vi "XY Graph Defer Owning VI Panel Update & Hide.vi"(6 "Defer Owning Panel Update":bool, 8 "error in (no error)":errorcluster, 11 "XY Graph Refnum in":refnum<vi>) -> (0 "error out":errorcluster, 3 "XY Graph Refnum out":refnum<vi>)   [LabVIEW 2019]
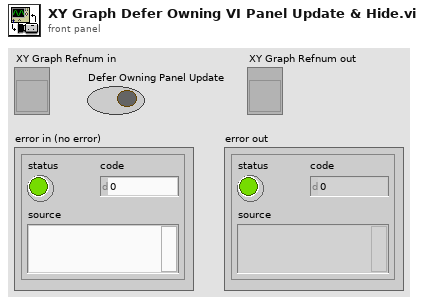
[diagram p1: front panel]
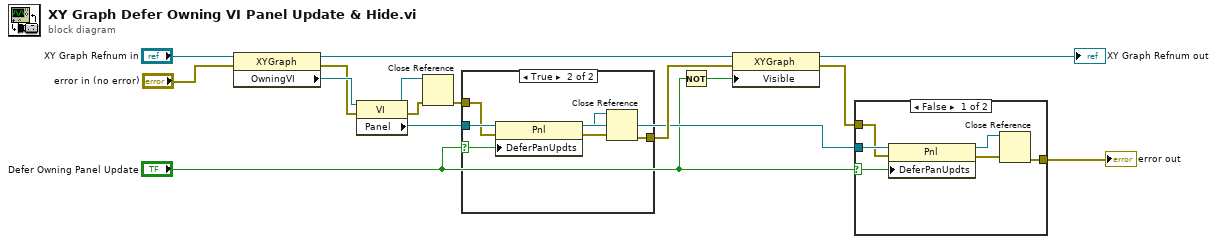
[diagram p0: block diagram]
diagram:
  n1 = property class="XYGraph"(reference="XY Graph Refnum in", error in="error in (no error)") -> (reference out=w13:refnum<vi>, error out=w3:errorcluster, "OwningVI"=w12:refnum<vi>)
  n2 = property class="VI"(reference=w12, error in=w3) -> (reference out=w11:refnum<vi>, error out=w10:errorcluster, "Panel"=w6:refnum<vi>)
  n3 = Close Reference(reference=w11, error in (no error)=w10) -> (error out=w7:errorcluster)
  n4 = case shown="True" "Defer Owning Panel Update" {
    selector: "Defer Owning Panel Update" -> [_ w18]
    tunnel: w6 -> [_ w22]
    tunnel: [w16 w19] -> w9
    tunnel: w7 -> [w16 w17]
    frame False {
    }
    frame True {
      n5 = property class="Pnl"(reference=w22, error in=w17, "DeferPanUpdts"=w18) -> (reference out=w20:refnum<vi>, error out=w21:errorcluster)
      n6 = Close Reference(reference=w20, error in (no error)=w21) -> (error out=w19:errorcluster)
    }
  }
  n7 = Not(x="Defer Owning Panel Update") -> (.not. x?=w8:bool)
  n8 = property class="XYGraph"(reference=w13, error in=w9, "Visible"=w8) -> (reference out=→"XY Graph Refnum out":refnum<vi>, error out=w4:errorcluster)
  n9 = case shown="False" "Defer Owning Panel Update" {
    selector: "Defer Owning Panel Update" -> [w25 _]
    tunnel: w6 -> [w28 _]
    tunnel: w4 -> [w24 w29]
    tunnel: [w23 w29] -> w2
    frame False {
      n10 = property class="Pnl"(reference=w28, error in=w24, "DeferPanUpdts"=w25) -> (reference out=w26:refnum<vi>, error out=w27:errorcluster)
      n11 = Close Reference(reference=w26, error in (no error)=w27) -> (error out=w23:errorcluster)
    }
    frame True {
    }
  }
  "error out" <- w2
